vi "CallPythonImageFunction.vi"(8 "error in (no error)":errorcluster, 9 "Function or Method Name":string="find_faces", 10 "Python Image Data in":u8[][][](array[numeric]), 11 "reference in":refnum<class "ImageFacialDetection.lvclass">) -> (0 "error out":errorcluster, 2 "Python Image Data out":u8[][][](array[numeric]), 3 "reference out":refnum<class "ImageFacialDetection.lvclass">)   [LabVIEW 2017, in "ImageFacialDetection.lvclass"]
doc: "uses the image classification in python with openCV to detect faces in an image using Haar Cascades"
uses:
  ImageFacialDetection.lvclass
  <vilib>/Enthought/Python Integration Toolkit/api/Unpack As Variant.vi
  <vilib>/Enthought/Python Integration Toolkit/Python Integration Toolkit.lvlib
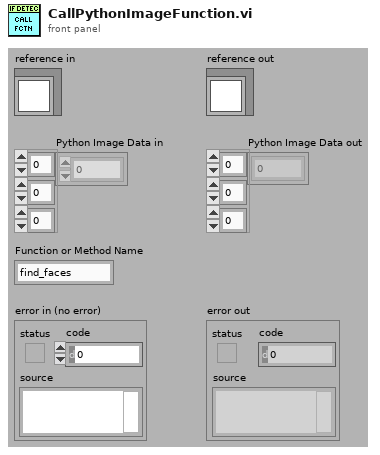
[diagram p1: front panel]
types:
  T1 = typedef "Python Integration Toolkit.lvlib/Session ID.ctl" = u64
  T2 = typedef "Python Integration Toolkit.lvlib/Python Objects.ctl" = variant
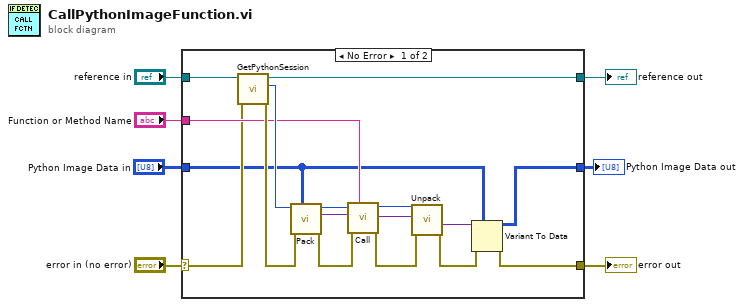
[diagram p0: block diagram]
diagram:
  n1 = case shown="No Error" "error in (no error)" {
    selector: "error in (no error)" -> [w10 w26]
    tunnel: [w13 w26] -> w6
    tunnel: [w23 w25] -> w4
    tunnel: "reference in" -> [w24 w25]
    tunnel: "Function or Method Name" -> [w11 _]
    tunnel: "Python Image Data in" -> [w8 _]
    tunnel: [w9 _] -> w1
    frame No Error {
      n2 = call "GetPythonSession.vi"("error in (no error)"=w10, "reference in"=w24) -> ("error out"=w21:errorcluster, "Python Session ID"=w22:T1, "reference out"=w23:refnum<class "ImageFacialDetection.lvclass">)  [unwired: 7 in]
      n3 = call <vilib>:"Pack.vi"("Argument"=w8, "error in (no error)"=w21, "Session ID"=w22) -> ("error out"=w18:errorcluster, "Python Object References Out"=w19:T2, "Session ID out"=w20:T1)  [unwired: 6 in]
      n4 = call <vilib>:"Call.vi"("Function or Method Name"=w11, "error in (no error)"=w18, "Python Object References In"=w19, "Session ID"=w20) -> ("error out"=w15:errorcluster, "Python Object References Out"=w16:T2, "Session ID out"=w17:T1)  [unwired: 5 in]
      n5 = call-poly <vilib>:"Unpack.vi"("error in (no error)"=w15, "Python Object References In"=w16, "Session ID"=w17) -> ("error out"=w14:errorcluster, "Value"=w12:variant)  [unwired: 5 in, 2 out]
      n6 = Variant To Data(error in=w14, type=w8, Variant=w12) -> (data=w9:u8[][][], error out=w13:errorcluster)
    }
    frame Error {
    }
  }
  "error out" <- w6
  "reference out" <- w4
  "Python Image Data out" <- w1
